vi "Compare Binary Strings.vi"(3 "Comparison String":string, 4 "MICS Data":string, 5 "Sequence Context":refnum<k7>) -> (0 "error out":errorcluster, 1 "x = y?":bool)   [LabVIEW 2010]
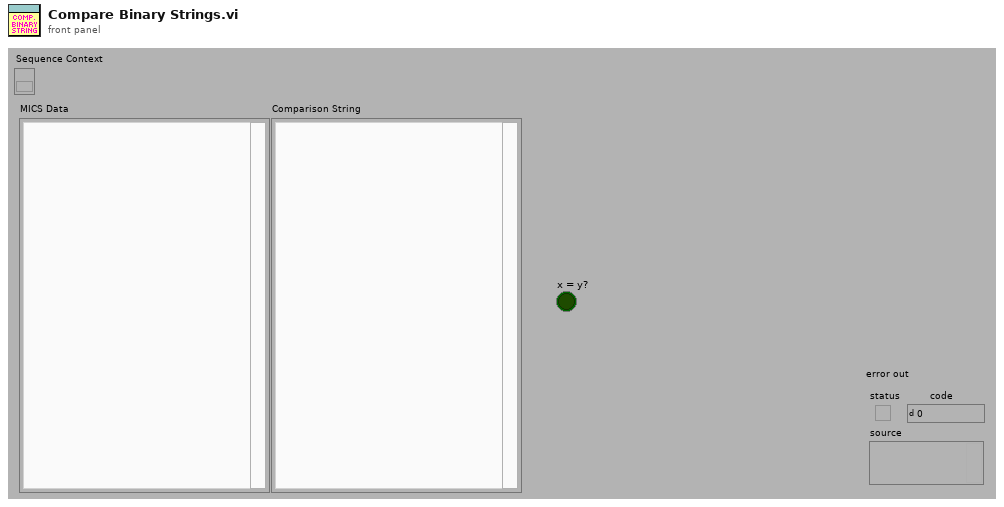
[diagram p1: front panel]
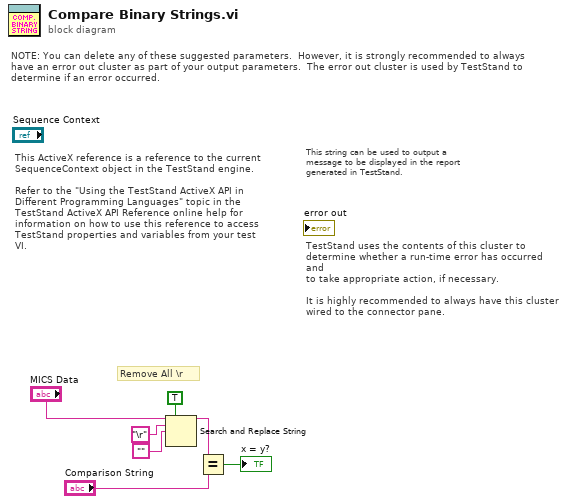
[diagram p0: block diagram]
diagram:
  # "Remove All \\r"
  # "TestStand uses the contents of this cluster to\ndetermine whether a run-time error has occurred and\nto take appropriate action, if necessary.\n\nIt is highly recommended to always have this cluster\nwired to the connector pane."
  # "This string can be used to output a\nmessage to be displayed in the report\ngenerated in TestStand."
  # "NOTE: You can delete any of these suggested parameters.  However, it is strongly recommended to always have an error out cluster as part of your output parameters.  The error out cluster is used by TestStand to determine if an error occurred."
  # "This ActiveX reference is a reference to the current\nSequenceContext object in the TestStand engine.\n\nRefer to the \"Using the TestStand ActiveX API in\nDifferent Programming Languages\" topic in the \nTestStand ActiveX API Reference online help for\ninformation on how to use this reference to access\nTestStand properties and variables from your test VI."
  n1 = Search and Replace String(replace all?=TRUE ("replace all? (F)"), input string="MICS Data", search string="\r", replace string="" ("search string")) -> (result string=w2:string)  [unwired: 4 in, 3 out]
  n2 = Equal?(x=w2, y="Comparison String") -> (x = y?=→"x = y?":bool)
